vi "SetVal.vi"(8 "error in (no error)":errorcluster caption="错误输入（无错误）", 10 "Vol":dbl, 11 "TH6402 输入":refnum<class "TH6402.lvclass">) -> (0 "error out":errorcluster caption="错误输出", 3 "TH6402 输出":refnum<class "TH6402.lvclass">)   [LabVIEW 2020, in "DP.lvlib" / "TH6402.lvclass"]
uses:
  TH6402.lvclass
  D:/Workspace/LabVIEW/LVProject/Class/LVDevClass/DP/root/DP.lvclass
  TH6402.lvclass/TH6402.ctl
  c727b7ae-e8f4-4648-a5f5-797d20be59b8.vi
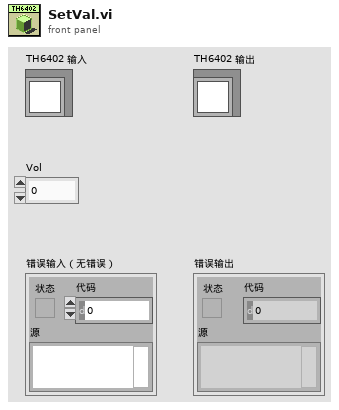
[diagram p1: front panel]
types:
  T1 = typedef "DP.lvlib/DP.lvclass/Function.ctl" = enum16{"CV", "CC"}
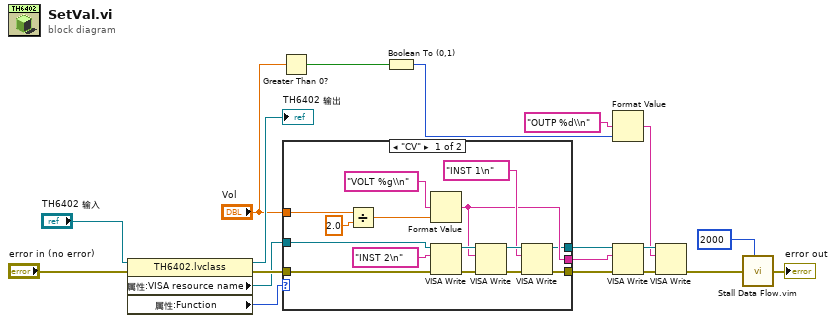
[diagram p0: block diagram]
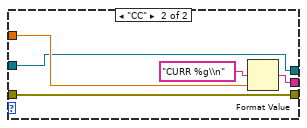
[diagram p2: hidden frame]
diagram:
  n1 = property class="TH6402.lvclass"(reference="TH6402 输入", error in="error in (no error)") -> (reference out=→"TH6402 输出":refnum<class "TH6402.lvclass">, error out=w11:errorcluster, "属性:VISA resource name"=w10:refnum<visa-resource-name>, "属性:Function"=w12:T1)
  n2 = Greater Than 0?(x="Vol") -> (x > 0?=w7:bool)
  n3 = case shown="\"CV\"" w12 {
    tunnel: w11 -> [w23 w37]
    tunnel: [w24 w38] -> w16
    tunnel: [w22 w37] -> w15
    tunnel: "Vol" -> [w34 w39]
    tunnel: w10 -> [w21 w35]
    tunnel: [w20 w35] -> w9
    frame "CV" {
      n4 = Divide(x=w34, y=2.0) -> (x/y=w25:dbl)
      n5 = Format Value(format string="VOLT %g\\n" ("格式字符串"), value (0)=w25) -> (output string=w24:string)  [unwired: 1 in]
      n6 = VISA Write(VISA resource name=w21, write buffer="INST 2\n" ("写入缓冲区"), error in (no error)=w23) -> (VISA resource name out=w31:refnum<visa-resource-name>, error out=w30:errorcluster)  [unwired: 1 out]
      n7 = VISA Write(VISA resource name=w31, write buffer=w24, error in (no error)=w30) -> (VISA resource name out=w33:refnum<visa-resource-name>, error out=w32:errorcluster)  [unwired: 1 out]
      n8 = VISA Write(VISA resource name=w33, write buffer="INST 1\n" ("写入缓冲区"), error in (no error)=w32) -> (VISA resource name out=w20:refnum<visa-resource-name>, error out=w22:errorcluster)  [unwired: 1 out]
    }
    frame "CC" {
      n9 = Format Value(format string="CURR %g\\n" ("格式字符串"), value (0)=w39) -> (output string=w38:string)  [unwired: 1 in]
    }
  }
  n10 = Boolean To (0,1)(Boolean=w7) -> (0, 1=w6:i16)
  n11 = Format Value(format string="OUTP %d\\n" ("格式字符串"), value (0)=w6) -> (output string=w5:string)  [unwired: 1 in]
  n12 = VISA Write(VISA resource name=w9, write buffer=w16, error in (no error)=w15) -> (VISA resource name out=w13:refnum<visa-resource-name>, error out=w4:errorcluster)  [unwired: 1 out]
  n13 = VISA Write(VISA resource name=w13, write buffer=w5, error in (no error)=w4) -> (error out=w2:errorcluster)  [unwired: 2 out]
  n14 = call "Stall Data Flow.vim"("value in"=w2, "milliseconds to wait"=u32 2000) -> ("value out"=→"error out":errorcluster)  [unwired: 1 out]
